vi "Tree_OutdentItem.vi"(8 "Error In":errorcluster, 10 "TagToOutdent":string, 11 "Tree Refnum":refnum<vi>) -> (0 "Error Out":errorcluster, 3 "Tree Refnum OUT":refnum<vi>)   [LabVIEW 2012]
doc: "SciScan 1.2 160622"
panel:
  in  "Tree":string(tree)
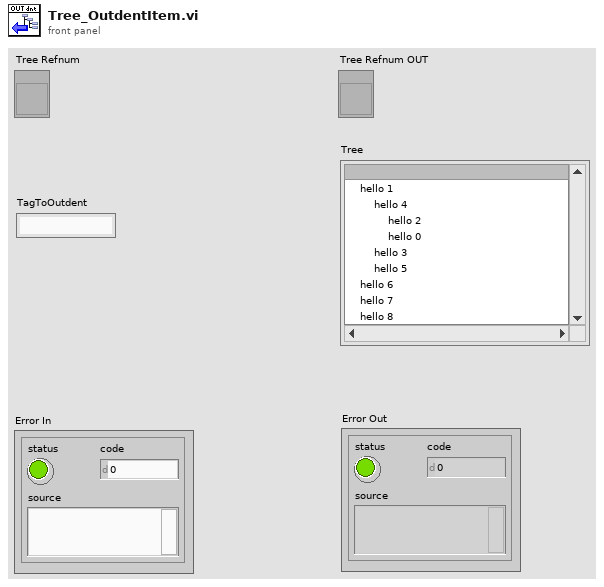
[diagram p1: front panel]
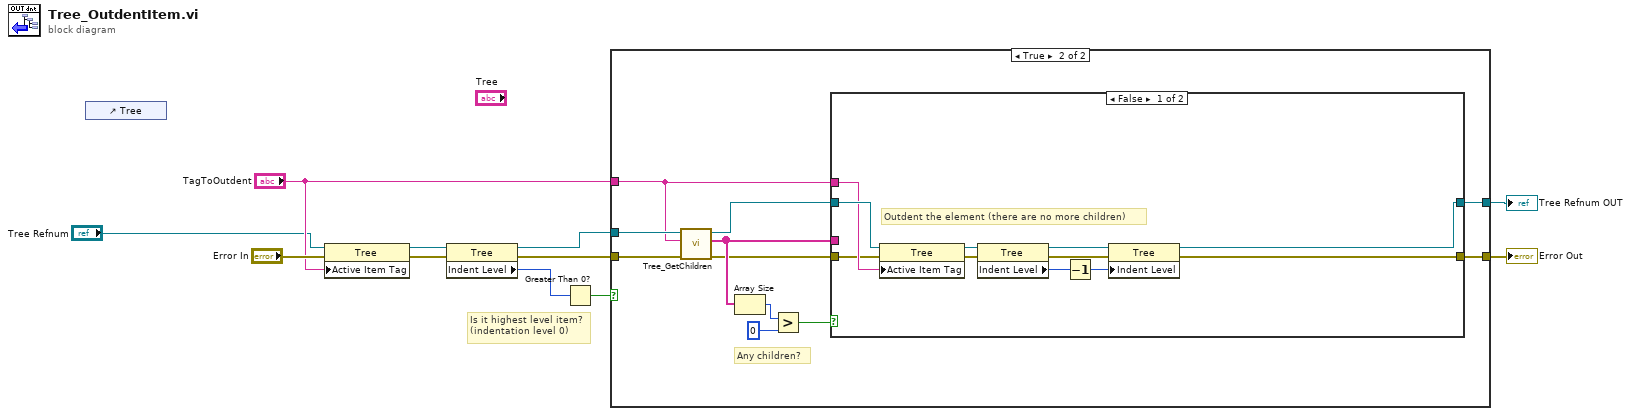
[diagram p0: block diagram]
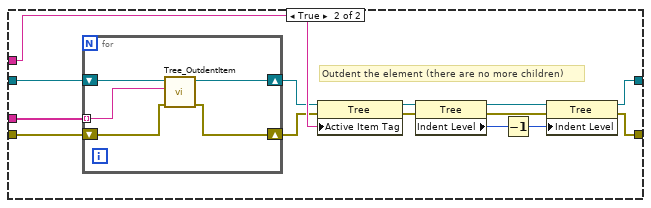
[diagram p3: hidden frame]
diagram:
  # "Is it highest level item?\n(indentation level 0)"
  n1 = control-ref of="Tree"() -> ()  [unwired: 1 out]
  n2 = property class="Tree"(reference="Tree Refnum", error in="Error In", "Active Item Tag"="TagToOutdent") -> (reference out=w8:refnum<vi>, error out=w9:errorcluster)
  n3 = property class="Tree"(reference=w8, error in=w9) -> (reference out=w7:refnum<vi>, error out=w6:errorcluster, "Indent Level"=w5:i32)
  n4 = Greater Than 0?(x=w5) -> (x > 0?=w4:bool)
  n5 = case shown="True" w4 {
    tunnel: w7 -> [w13 w23]
    tunnel: "TagToOutdent" -> [_ w18]
    tunnel: [w13 w17] -> w11
    tunnel: w6 -> [w12 w16]
    tunnel: [w12 w14] -> w10
    frame False {
    }
    frame True {
      # "Any children?"
      n6 = call "Tree_GetChildren.vi"("Error In"=w16, "Parent Tag"=w18, "Tree Refnum IN"=w23) -> ("Error Out"=w15:errorcluster, "Children Tags"=w20:string[], "Tree Refnum OUT"=w24:refnum<vi>)  [unwired: 6 in]
      n7 = Array Size(array=w20) -> (size(s)=w22:i32)
      n8 = Greater?(x=w22, y=0) -> (0:w19:bool)
      n9 = case shown="False" w19 {
        tunnel: w24 -> [w31 w49]
        tunnel: w20 -> [_ w48]
        tunnel: w18 -> [w30 w40]
        tunnel: [w29 w36] -> w17
        tunnel: w15 -> [w27 w47]
        tunnel: [w28 w37] -> w14
        frame False {
          # "Outdent the element (there are no more children)"
          n10 = property class="Tree"(reference=w31, error in=w27, "Active Item Tag"=w30) -> (reference out=w25:refnum<vi>, error out=w35:errorcluster)
          n11 = property class="Tree"(reference=w25, error in=w35) -> (reference out=w26:refnum<vi>, error out=w34:errorcluster, "Indent Level"=w33:i32)
          n12 = Decrement(x=w33) -> (x-1=w32:i32)
          n13 = property class="Tree"(reference=w26, error in=w34, "Indent Level"=w32) -> (reference out=w29:refnum<vi>, error out=w28:errorcluster)
        }
        frame True {
          # "Outdent the element (there are no more children)"
          n14 = for {
            tunnel: w48 -> [w54] mode=indexing
            shift-right: [w52] -> w39
            shift-left: w49 -> [w53]
            shift-right: [w50] -> w38
            shift-left: w47 -> [w51]
            n15 = call "Tree_OutdentItem.vi"("Error In"=w51, "TagToOutdent"=w54, "Tree Refnum"=w53) -> ("Error Out"=w50:errorcluster, "Tree Refnum OUT"=w52:refnum<vi>)  [unwired: 7 in]
          }
          n16 = property class="Tree"(reference=w39, error in=w38, "Active Item Tag"=w40) -> (reference out=w41:refnum<vi>, error out=w46:errorcluster)
          n17 = property class="Tree"(reference=w41, error in=w46) -> (reference out=w42:refnum<vi>, error out=w45:errorcluster, "Indent Level"=w44:i32)
          n18 = Decrement(x=w44) -> (x-1=w43:i32)
          n19 = property class="Tree"(reference=w42, error in=w45, "Indent Level"=w43) -> (reference out=w36:refnum<vi>, error out=w37:errorcluster)
        }
      }
    }
  }
  "Error Out" <- w10
  "Tree Refnum OUT" <- w11
